vi "Read Pull_in.vi"(8 "error in (no error)":errorcluster, 11 "EVI 79 in":refnum<class "EVI 79.lvclass">) -> (0 "error out":errorcluster, 2 "Pull_in":T1={"V"=0.0, "I"=0.5, "V_increased"=9.0, "V_perturb"=0.01, "Plunger_Threshold"=0.01, "V_MAX"=1.0}, 3 "EVI 79 out":refnum<class "EVI 79.lvclass">)   [LabVIEW 2025, in "EVI 79.lvclass"]
uses:
  EVI 79.lvclass
  EVI 79.lvclass/EVI 79.ctl
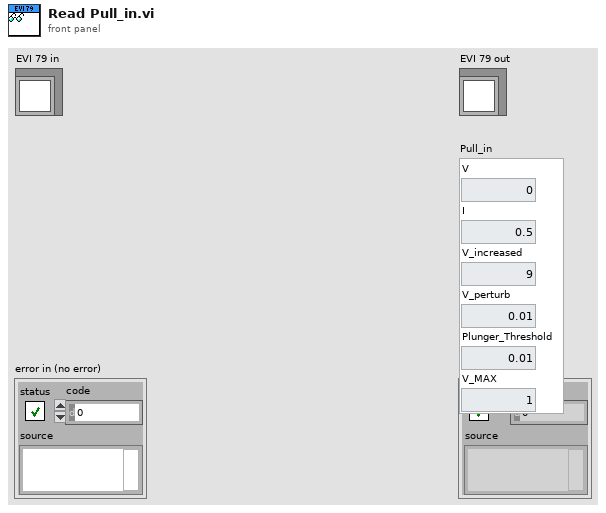
[diagram p1: front panel]
types:
  T1 = cluster{"V":dbl, "I":dbl, "V_increased":dbl, "V_perturb":dbl, "Plunger_Threshold":dbl, "V_MAX":dbl}
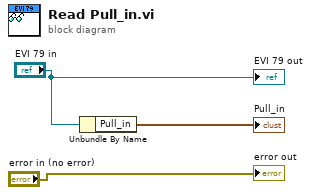
[diagram p0: block diagram]
diagram:
  n1 = Unbundle By Name("EVI 79 in") -> ("Pull_in"=→"Pull_in":T1)
  "error out" <- "error in (no error)"
  "EVI 79 out" <- "EVI 79 in"
